vi "_RS485 Driver.vi"(0 "RS485 Settings":T1=[{"Clock Source"=TRUE, "Clock Speed (Hz)"=0}, {"Clock Source"=TRUE, "Clock Speed (Hz)"=0}, {"Clock Source"=TRUE, "Clock Speed (Hz)"=0}, {"Clock Source"=TRUE, "Clock Speed (Hz)"=0}], 5 "Error IN":errorcluster, 8 "Action":T3) -> (14 "Serial Data Out":T2, 16 "Beat":bool, 19 "Error OUT":errorcluster)   [LabVIEW 2011]
uses:
  Controls/Serial_Action_Enum.ctl
  Controls/Serial Data Cluster.ctl
  Utilities/Program Control/RS485 Settings Top Level.ctl
  <vilib>/Utility/error.llb/Error Cluster From Error Code.vi
  <vilib>/rvi/errors/niLvFpgaAdjustHostInterfaceError.vi
  <vilib>/FPGAPlugInAG/sbRIO-9606/niLvFpga_Close_sbRIO-9606.vi
  <vilib>/rvi/interface/nirviReadWriteControl/nirviReadWriteControl.xnode
  FPGA Bitfiles/JAGM_FPGATarget_FPGAMain_A31A659D.lvbitx
  FPGA Source/FPGA Main.vi
  <vilib>/rvi/interface/nirviCloseFPGA/nirviCloseFPGA.xnode
  NiFpgaLv.dll
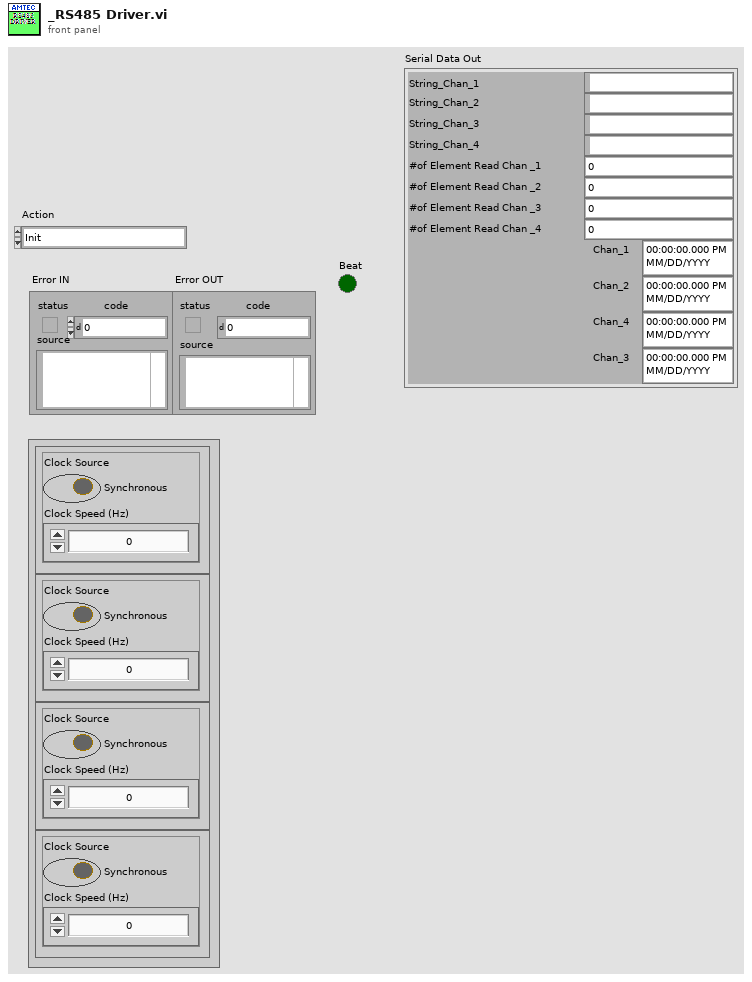
[diagram p1: front panel]
types:
  T1 = typedef "RS485 Settings Top Level.ctl" = cluster{"Clock Source":bool, "Clock Speed (Hz)":u32}[]
  T2 = typedef "Serial Data Cluster.ctl" = cluster{"String_Chan_1":string, "String_Chan_2":string, "String_Chan_3":string, "String_Chan_4":string, "#of Element Read Chan _1":i32, "#of Element Read Chan _2":i32, "#of Element Read Chan _3":i32, "#of Element Read Chan _4":i32, "Chan_1":timestamp, "Chan_2":timestamp, "Chan_3":timestamp, "Chan_4":timestamp}
  T3 = typedef "Serial_Action_Enum.ctl" = enum16{"Init", "Status", "Close", "Read All Chan", "Set Read Start Bit", "Clear Read Start Bit", "Read Beat", "Set RS485 Settings", "Close Ref"}
  T4 = cluster{"Data Bit(8)":i32, "Stop Bit":u16, "Baud Rate":u32, "Invert Polarity?":bool, " Mode":bool}[]
  T5 = cluster{"Data Bit(8)":i32, "Stop Bit":u16, "Baud Rate":u32, "Invert Polarity?":bool, " Mode":bool}
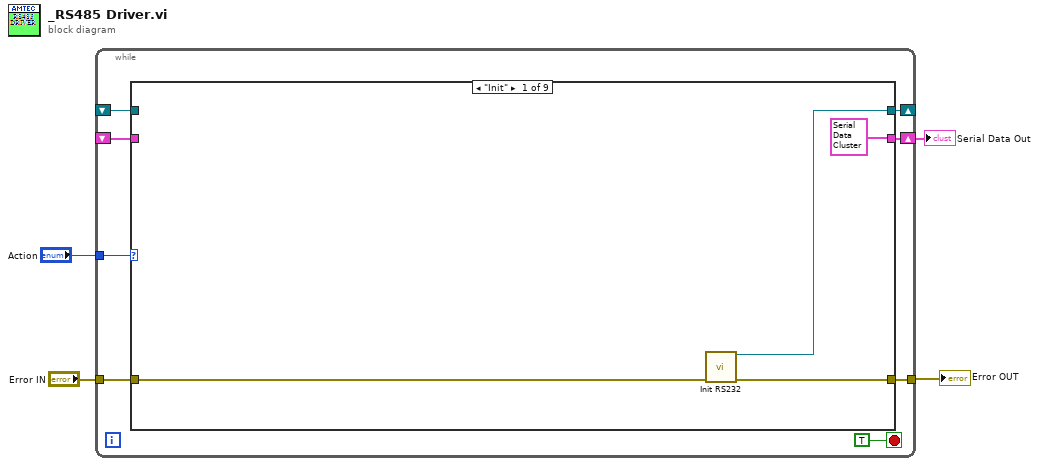
[diagram p0: block diagram]
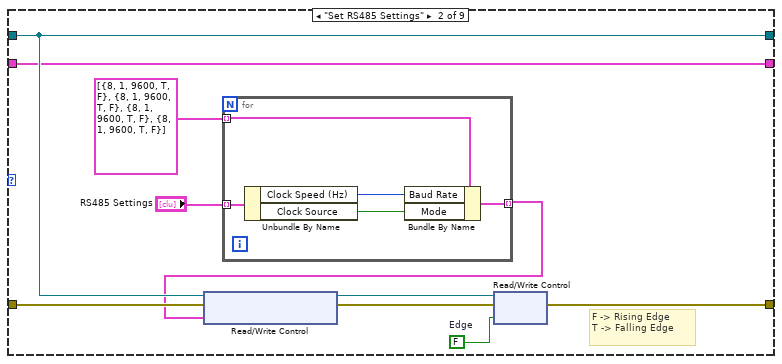
[diagram p2: hidden frame]
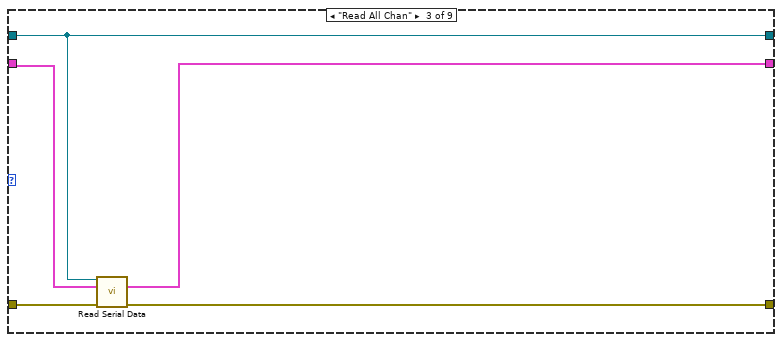
[diagram p3: hidden frame]
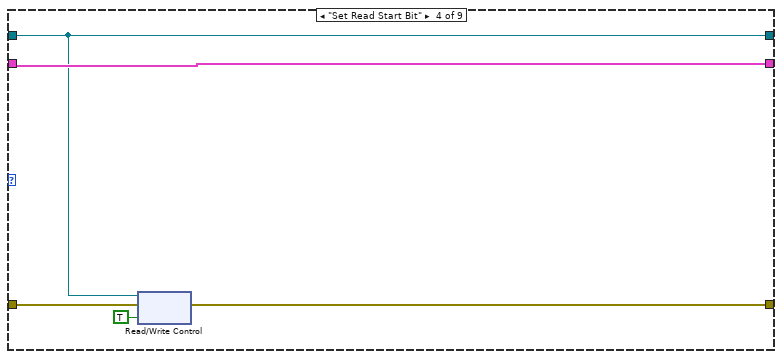
[diagram p4: hidden frame]
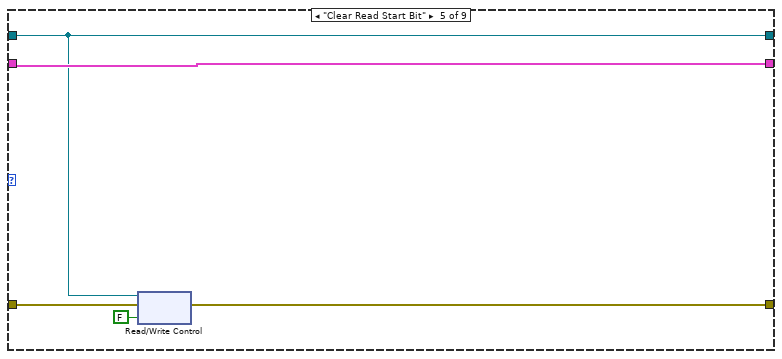
[diagram p5: hidden frame]
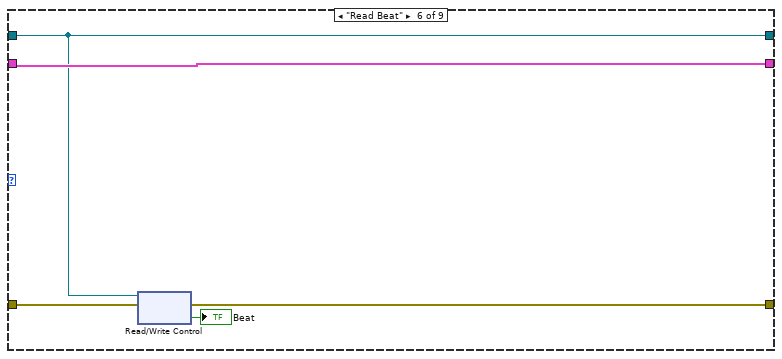
[diagram p6: hidden frame]
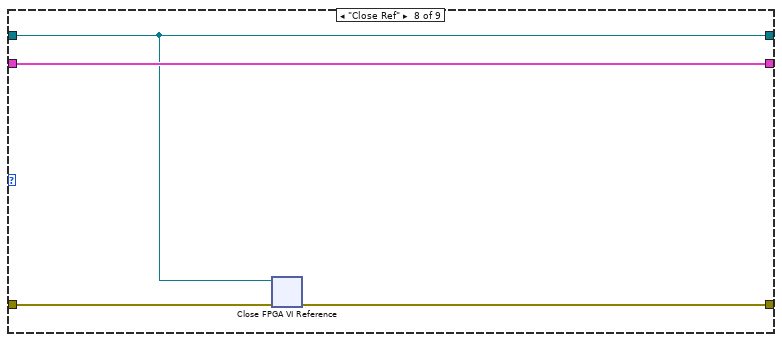
[diagram p8: hidden frame]
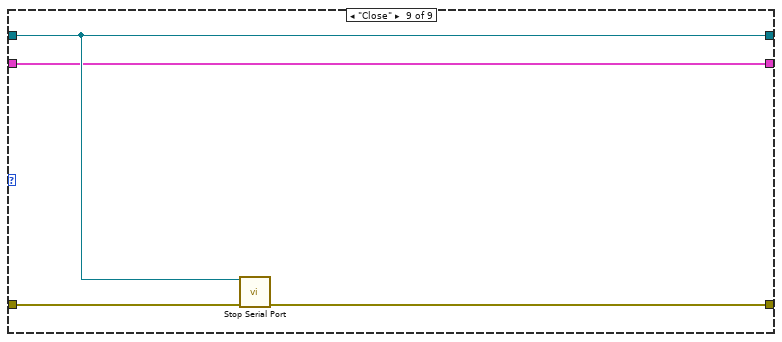
[diagram p9: hidden frame]
diagram:
  n1 = while {
    tunnel: "Action" -> [w11]
    tunnel: "Error IN" -> [w10]
    tunnel: [w9] -> w3
    shift-right: [w8] -> _
    shift-left: _ -> [w7]
    shift-right: [w6] -> w1
    shift-left: _ -> [w5]
    stop <- TRUE stop-if-true
    n2 = case shown="\"Init\"" w11 {
      tunnel: w10 -> [w16 w22 w36 w38 w43 w49 w54 w57 w62]
      tunnel: [w15 w20 w35 w37 w42 w48 w54 w56 w61] -> w9
      tunnel: [w14 w23 w34 w39 w44 w50 w53 w55 w60] -> w8
      tunnel: w7 -> [_ w23 w34 w39 w44 w50 w53 w55 w60]
      tunnel: [T2 {"String_Chan_1"="", "String_Chan_2"="", "String_Chan_3"="", "String_Chan_4"="", "#of Element Read Chan _1"=0, "#of Element Read Chan _2"=0, "#of Element Read Chan _3"=0, "#of Element Read Chan _4"=0, "Chan_1"=timestamp(0 s since 1904-01-01), "Chan_2"=timestamp(0 s since 1904-01-01), "Chan_3"=timestamp(0 s since 1904-01-01), "Chan_4"=timestamp(0 s since 1904-01-01)} ("Serial Data Out") w21 w33 w41 w46 w51 w52 w58 w59] -> w6
      tunnel: w5 -> [_ w21 w32 w41 w46 w51 w52 w58 w59]
      frame "Init" {
        n3 = call "Init RS232.vi"("Error IN"=w16) -> ("FPGA Main Reference Out"=w14:refnum<k20>, "error out"=w15:errorcluster)  [unwired: 13 in]
      }
      frame "Set RS485 Settings" {
        w24 = FALSE  # Edge
        # "F -> Rising Edge\nT -> Falling Edge"
        n4 = for {
          tunnel: "RS485 Settings" -> [w31] mode=indexing
          tunnel: T4 [{"Data Bit(8)"=8, "Stop Bit"=1, "Baud Rate"=9600, "Invert Polarity?"=TRUE, " Mode"=FALSE}, {"Data Bit(8)"=8, "Stop Bit"=1, "Baud Rate"=9600, "Invert Polarity?"=TRUE, " Mode"=FALSE}, {"Data Bit(8)"=8, "Stop Bit"=1, "Baud Rate"=9600, "Invert Polarity?"=TRUE, " Mode"=FALSE}, {"Data Bit(8)"=8, "Stop Bit"=1, "Baud Rate"=9600, "Invert Polarity?"=TRUE, " Mode"=FALSE}] ("Port Settings - 4 Chan") -> [w30] mode=indexing
          tunnel: [w27] -> w17 mode=indexing
          n5 = Unbundle By Name(w31) -> ("Clock Speed (Hz)"=w29:u32, "Clock Source"=w28:bool)
          n6 = Bundle By Name(cluster=w30, "Baud Rate"=w29, "Mode"=w28) -> (w27:T5)
        }
        n7 = xnode "Read/Write Control"("FPGA VI Reference In"=w23, "error in"=w22, "Port Settings - 4 Chan"=w17) -> ("FPGA VI Reference Out"=w26:refnum<k20>, "error out"=w25:errorcluster)
        n8 = xnode "Read/Write Control"("FPGA VI Reference In"=w26, "error in"=w25, "Edge"=w24) -> ("error out"=w20:errorcluster)  [unwired: 1 out]
      }
      frame "Read All Chan" {
        n9 = call "Read Serial Data.vi"("FPGA Main IN"=w34, "Serial Data IN"=w32, "Error IN"=w36) -> ("Serial Data Out"=w33:T2, "Error OUT"=w35:errorcluster)  [unwired: 10 in, 1 out]
      }
      frame "Set Read Start Bit" {
        n10 = xnode "Read/Write Control"("FPGA VI Reference In"=w39, "error in"=w38, "Read"=TRUE) -> ("error out"=w37:errorcluster)  [unwired: 1 out]
      }
      frame "Clear Read Start Bit" {
        n11 = xnode "Read/Write Control"("FPGA VI Reference In"=w44, "error in"=w43, "Read"=FALSE) -> ("error out"=w42:errorcluster)  [unwired: 1 out]
      }
      frame "Read Beat" {
        n12 = xnode "Read/Write Control"("FPGA VI Reference In"=w50, "error in"=w49) -> ("error out"=w48:errorcluster, "Beat"=→"Beat":bool)  [unwired: 1 out]
      }
      frame "Status", Default {
      }
      frame "Close Ref" {
        n13 = xnode "Close FPGA VI Reference"("FPGA VI Reference In"=w55, "error in"=w57) -> ("error out"=w56:errorcluster)
      }
      frame "Close" {
        n14 = call "Stop Serial Port.vi"("FPGA Main Ref"=w60, "Error IN"=w62) -> ("Error OUT"=w61:errorcluster)  [unwired: 13 in]
      }
    }
  }
  "Error OUT" <- w3
  "Serial Data Out" <- w1
